vi "ActionVIOnCompile.vi"(8 "error in (no error)":errorcluster, 11 "Device Item Ref in":T1 format="%.0x") -> (0 "error out":errorcluster)   [LabVIEW 2019, in "OPC UA Client Addon System Explorer.lvlib"]
uses:
  OPC UA Client Addon System Explorer.lvlib
  <vilib>/NI VeriStand/Custom Device API/Custom Device Item Ref.ctl
  Addon Shared/Types/Tag.WriteProperties.Info.ctl
  <vilib>/NI VeriStand/Custom Device API/Data Reference.ctl
  Addon Shared/Types/Compiled.Settings.ctl
  Addon Shared/Types/OPCConnection.Properties.ctl
  Addon Shared/Types/Poll.ListProperties.ctl
  Addon Shared/Types/Tags.ReadWriteRefs.ctl
  <vilib>/NI VeriStand/Custom Device API/Custom Device Target Type.ctl
  <vilib>/NI VeriStand/Custom Device API/Data Access Type.ctl
  Addon Shared/Types/DataRefs.Location.ctl
  Addon Shared/SubVIs/Constants.vi
  <vilib>/NI VeriStand/Custom Device API/NI VeriStand - Get Item Property.vi
  <vilib>/NI VeriStand/Custom Device API/Get Item Property (String).vi
  <vilib>/NI VeriStand/Custom Device API/Get Item Property (U16).vi
  <vilib>/NI VeriStand/Custom Device API/Get Item Property (Dependent File).vi
  <vilib>/NI VeriStand/Custom Device API/Set Item Property (String).vi
  <vilib>/NI VeriStand/Custom Device API/Set Item Property (U16).vi
  <vilib>/Utility/libraryn.llb/Get File Extension.vi
  <vilib>/Utility/MD5Checksum.llb/MD5Checksum File.vi
  <vilib>/NI VeriStand/Custom Device API/Set Item Property (Dependent File).vi
  <vilib>/Utility/libraryn.llb/Check if File or Folder Exists.vi
  <vilib>/NI VeriStand/Custom Device API/NI VeriStand - Remove Item Property.vi
  <vilib>/NI VeriStand/Custom Device Tools/Custom Device Utility Library/NI VeriStand - Search for Item by GUID.vi
  <vilib>/NI VeriStand/Custom Device Tools/Custom Device Utility Library/NI VeriStand - Search for All Items by GUID.vi
  <vilib>/NI VeriStand/Custom Device API/Get Item Property (Dependent Node Pointer).vi
  <vilib>/NI VeriStand/Custom Device API/Set Item Property (U32).vi
  <vilib>/NI VeriStand/Custom Device API/Get Item Property (U32).vi
  <vilib>/NI VeriStand/Custom Device Tools/Custom Device Utility Library/NI VeriStand - Search for Item by Name.vi
  <vilib>/NI VeriStand/Custom Device API/Set Item Property (Variant).vi
  <vilib>/NI VeriStand/Custom Device Tools/Custom Device Utility Library/Custom Device Utility Library.lvlib
  Addon Shared/OPC UA Client Addon Shared.lvlib
  <vilib>/NI VeriStand/Custom Device API/Custom Device API.lvlib
  <vilib>/NI/NIVS Inline Async API/_Data Access System Explorer/Data Access System Explorer.lvlib
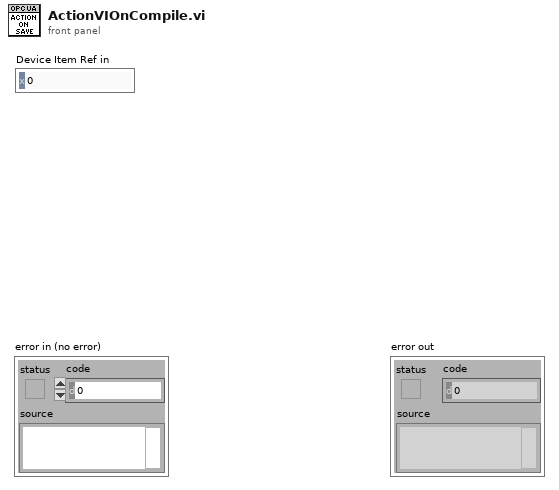
[diagram p1: front panel]
types:
  T1 = typedef "Custom Device API.lvlib/Custom Device Item Ref.ctl" = u64
  T2 = enum16{"Output/Write", "Input/Read", "Input/ReadWrite"}
  T3 = cluster{"Name":string, "Type":enum16{"Output/Write", "Input/Read", "Input/ReadWrite"}, "VS Refs":T1[]}
  T4 = typedef "OPC UA Client Addon Shared.lvlib/Tag.WriteProperties.Info.ctl" = cluster{"Path":string, "Offset":i32, "Length":i32, "DataType":u32}
  T5 = typedef "Custom Device API.lvlib/Data Reference.ctl" = i32
  T6 = typedef "OPC UA Client Addon Shared.lvlib/Compiled.Settings.ctl" = cluster{"Connection.Properties":T7, "PollEngine.Settings":T8[], "LUT":variant, "Write Locations":T4[], "TotalTags":u32, "Data Refs":T9, "Target Type":T10}
  T7 = typedef "OPC UA Client Addon Shared.lvlib/OPCConnection.Properties.ctl" = cluster{"Server IP Address":string, "Server Port":u16, "Message Mode":enum16{"None", "Sign", "Sign and Encrypt"}, "Security":enum16{"Basic256", "Basic128Rsa15"}, "User Name":string, "Password":string, "Client Certificate":path, "Server Certificate":path, "Server Certificate (RT)":path, "Client Certificate (RT)":path}
  T8 = typedef "OPC UA Client Addon Shared.lvlib/Poll.ListProperties.ctl" = cluster{"Poll Rate":dbl, "Tags":string[]}
  T9 = typedef "OPC UA Client Addon Shared.lvlib/Tags.ReadWriteRefs.ctl" = cluster{"Read Refs":T5[], "Read Values":dbl[], "Read?":bool[], "Access":enum8{"Null", "Read", "Write", "Read&Write"}[], "Write Refs":T5[], "Write Values":dbl[], "Write?":bool[], "Write Only Location":u32, "Write? Reset":bool[]}
  T10 = typedef "Custom Device API.lvlib/Custom Device Target Type.ctl" = enum16{"PharLap", "VxWorks", "Windows", "Linux_32_ARM", "Linux_x64"}
  T11 = typedef "Custom Device API.lvlib/Data Access Type.ctl" = enum16{"Read", "Write"}
  T12 = typedef "OPC UA Client Addon Shared.lvlib/DataRefs.Location.ctl" = cluster{"Offset":i32, "Length":i32}
  T13 = typedef "OPC UA Client Addon Shared.lvlib/Tag.Settings.ctl" = cluster{"TagPath":string, "DataType":u32, "DataAccess":u32}
  T14 = cluster{"Name":string, "Type":enum16{"Output/Write", "Input/Read", "Input/ReadWrite"}, "VS Refs":T1[]}[]
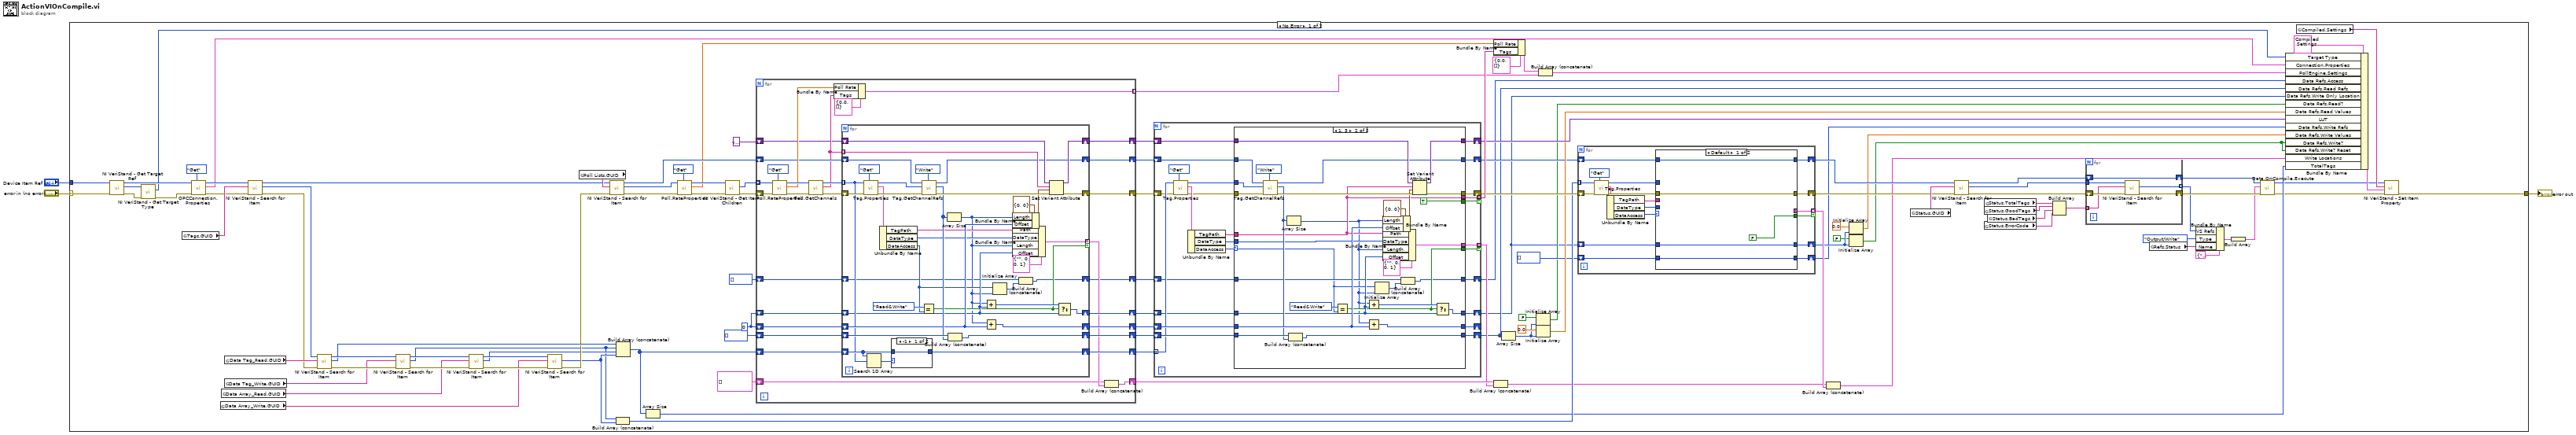
[diagram p0: block diagram]
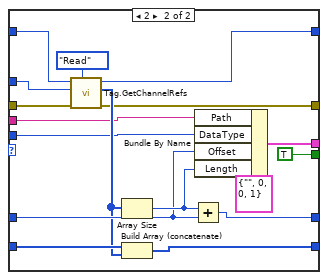
[diagram p2: hidden frame]
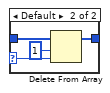
[diagram p4: hidden frame]
diagram:
  n1 = case shown="No Error" "error in (no error)" {
    selector: "error in (no error)" -> [w8 w295]
    tunnel: [w82 w295] -> w2
    tunnel: "Device Item Ref in" -> [w7 _]
    frame No Error {
      w43 = 0
      n2 = call <vilib>:"NI VeriStand - Get Target Ref.vi"("error in"=w8, "Item Ref in"=w7) -> ("error out"=w9:errorcluster, "Target Ref"=w10:T1, "Item Ref out"=w6:T1)  [unwired: 6 in, 1 out]
      n3 = call <vilib>:"NI VeriStand - Get Target Type.vi"("error in (no error)"=w9, "Item Ref in"=w10) -> ("error out"=w5:errorcluster, "Target Type"=w4:T10)  [unwired: 7 in, 1 out]
      n4 = global read "Constants.vi" "Tags.GUID"() -> (w103:string)
      n5 = call "OPCConnection.Properties.vi"("Action"=enum8{"Get", "Set"}."Get", "error in (no error)"=w5, "Item Ref in"=w6) -> ("error out"=w102:errorcluster, "Connection.Properties"=w83:T7, "Item Ref out"=w84:T1)  [unwired: 6 in]
      n6 = global read "Constants.vi" "Data Array_Write.GUID"() -> (w62:string)
      n7 = global read "Constants.vi" "Data Array_Read.GUID"() -> (w63:string)
      n8 = global read "Constants.vi" "Data Tag_Write.GUID"() -> (w96:string)
      n9 = global read "Constants.vi" "Data Tag_Read.GUID"() -> (w99:string)
      n10 = call-poly <vilib>:"NI VeriStand - Search for Item.vi"("error in"=w102, "Item GUID"=w103, "Section Ref in"=w84) -> ("error out"=w95:errorcluster, "Item Ref"=w100:T1, "Section Ref out"=w101:T1)  [unwired: 5 in, 1 out]
      n11 = call-poly <vilib>:"NI VeriStand - Search for Item.vi"("error in"=w95, "Item GUID"=w99, "Section Ref in"=w100) -> ("error out"=w97:errorcluster, "Item Refs"=w94:T1[], "Section Ref out"=w98:T1)  [unwired: 5 in, 1 out]
      n12 = call-poly <vilib>:"NI VeriStand - Search for Item.vi"("error in"=w97, "Item GUID"=w96, "Section Ref in"=w98) -> ("error out"=w66:errorcluster, "Item Refs"=w59:T1[], "Section Ref out"=w64:T1)  [unwired: 5 in, 1 out]
      n13 = call-poly <vilib>:"NI VeriStand - Search for Item.vi"("error in"=w66, "Item GUID"=w63, "Section Ref in"=w64) -> ("error out"=w68:errorcluster, "Item Refs"=w61:T1[], "Section Ref out"=w67:T1)  [unwired: 5 in, 1 out]
      n14 = call-poly <vilib>:"NI VeriStand - Search for Item.vi"("error in"=w68, "Item GUID"=w62, "Section Ref in"=w67) -> ("error out"=w65:errorcluster, "Item Refs"=w60:T1[])  [unwired: 5 in, 2 out]
      n15 = global read "Constants.vi" "Poll Lists.GUID"() -> (w111:string)
      n16 = call-poly <vilib>:"NI VeriStand - Search for Item.vi"("error in"=w65, "Item GUID"=w111, "Section Ref in"=w101) -> ("error out"=w110:errorcluster, "Item Ref"=w109:T1, "Section Ref out"=w93:T1)  [unwired: 5 in, 1 out]
      n17 = Build Array (concatenate)(w59, w60) -> (w57:T1[])
      n18 = Build Array (concatenate)(w94, w59, w61, w60) -> (w55:T1[])
      n19 = Array Size(array=w55) -> (size(s)=w54:i32)
      n20 = call "Poll.RateProperties.vi"("Action"=enum8{"Get", "Set"}."Get", "error in (no error)"=w110, "Item Ref in"=w109) -> ("error out"=w107:errorcluster, "Poll Rate"=w87:dbl, "Item Ref out"=w106:T1)  [unwired: 6 in]
      n21 = call <vilib>:"NI VeriStand - Get Item Children.vi"("error in (no error)"=w107, "Item Ref in"=w106) -> ("error out"=w105:errorcluster, "Child Refs"=w104:T1[])  [unwired: 6 in, 2 out]
      n22 = for {
        tunnel: w104 -> [w249] mode=indexing
        shift-right: [w245] -> w90
        shift-left: w55 -> [w246]
        shift-right: [w241] -> w89
        shift-left: w105 -> [w250]
        tunnel: [w238] -> w85 mode=indexing
        shift-right: [w236] -> w91
        shift-left: w93 -> [w240]
        shift-right: [w234] -> w70
        shift-left: variant ("variant") -> [w235]
        shift-right: [w232] -> w51
        shift-left: T5[] [] ("Array") -> [w233]
        shift-right: [w230] -> w50
        shift-left: w43 -> [w231]
        shift-right: [w228] -> w41
        shift-left: w43 -> [w229]
        shift-right: [w226] -> w40
        shift-left: T4[] [] -> [w225]
        shift-right: [w224] -> w29
        shift-left: u32[] [] -> [w223]
        n23 = call "Poll.RateProperties.vi"("Action"=enum8{"Get", "Set"}."Get", "error in (no error)"=w250, "Item Ref in"=w249) -> ("error out"=w248:errorcluster, "Poll Rate"=w244:dbl, "Item Ref out"=w247:T1)  [unwired: 6 in]
        n24 = call "Poll.GetChannels.vi"("error in (no error)"=w248, "Node Ptr"=w247) -> ("error out"=w242:errorcluster, "Tags"=w239:string[], "Refs"=w243:T1[])  [unwired: 7 in]
        n25 = Bundle By Name(cluster=T8 {"Poll Rate"=0.0, "Tags"=[]}, "Poll Rate"=w244, "Tags"=w239) -> (w238:T8)
        n26 = for {
          tunnel: w243 -> [w270] mode=indexing
          shift-right: [w288] -> w245
          shift-left: w246 -> [w287]
          shift-right: [w284] -> w241
          shift-left: w242 -> [w272]
          shift-right: [w281] -> w234
          shift-left: w235 -> [w283]
          tunnel: w239 -> [w282] mode=indexing
          shift-right: [w280] -> w236
          shift-left: w240 -> [w285]
          shift-right: [w278] -> w232
          shift-left: w233 -> [w279]
          shift-right: [w276] -> w230
          shift-left: w231 -> [w274]
          shift-right: [w260] -> w228
          shift-left: w229 -> [w261]
          tunnel: [w259] -> w227 mode=indexing if=w258
          shift-right: [w253] -> w224
          shift-left: w223 -> [w252]
          n27 = call "Tag.Properties.vi"("Action"=enum8{"Get", "Set"}."Get", "error in (no error)"=w272, "Section Ref in"=w270) -> ("error out"=w271:errorcluster, "Channel Settings"=w266:T13, "Item Ref out"=w269:T1)  [unwired: 6 in]
          n28 = Search 1D Array(1D array=w287, element=w270) -> (index of element=w289:i32)  [unwired: 1 in]
          n29 = Unbundle By Name(w266) -> ("TagPath"=w265:string, "DataType"=w264:u32, "DataAccess"=w256:u32)
          n30 = case shown="-1" w289 {
            selector: w289 -> [_ w293]
            tunnel: [w290 w291] -> w288
            tunnel: w287 -> [w290 w294]
            frame -1 {
            }
            frame Default {
              n31 = Delete From Array(array=w294, length=1, index=w293) -> (array with subset deleted=w291:T1[])  [unwired: 1 out]
            }
          }
          n32 = Equal?(x=enum16{"Null", "Read", "Write", "Read&Write"}."Read&Write" ("access"), y=w256) -> (x = y?=w258:bool)
          n33 = call "Tag.GetChannelRefs.vi"("Access"=Data_Access_Type."Write", "error in (no error)"=w271, "Dependent Node Ref"=w269, "Section Ref in"=w285) -> ("error out"=w286:errorcluster, "Array"=w277:T5[], "Section Ref out"=w280:T1)  [unwired: 5 in]
          n34 = Array Size(array=w277) -> (size(s)=w255:i32)
          n35 = Build Array (concatenate)(w279, w277) -> (w278:T5[])
          n36 = Add(x=w255, y=w261) -> (x+y=w262:i32)
          n37 = Add(x=w255, y=w274) -> (x+y=w276:i32)
          n38 = Initialize Array(w256, w255) -> (w254:u32[])
          n39 = Bundle By Name(cluster=T12 {"Offset"=0, "Length"=0}, "Length"=w255, "Offset"=w274) -> (w273:T12)
          n40 = Bundle By Name(cluster=T4 {"Path"="", "Offset"=0, "Length"=0, "DataType"=1} ("WriteData.Info"), "Path"=w265, "DataType"=w264, "Length"=w255, "Offset"=w261) -> (w259:T4)
          n41 = Build Array (concatenate)(w252, w254) -> (w253:u32[])
          n42 = Set Variant Attribute(Variant=w283, name=w282, value=w273, error in=w286) -> (Variant out=w281:variant, error out=w284:errorcluster)  [unwired: 1 out]
          n43 = Select(t=w262, s=w258, f=w261) -> (s? t:f=w260:i32)
        }
        n44 = Build Array (concatenate)(w225, w227) -> (w226:T4[])
      }
      n45 = for {
        shift-right: [w183] -> w58
        shift-left: w89 -> [w172]
        shift-right: [w181] -> w69
        shift-left: w70 -> [w182]
        tunnel: w90 -> [w174] mode=indexing
        shift-right: [w180] -> w47
        shift-left: w91 -> [w184]
        tunnel: [w166] -> w88 mode=indexing if=w179
        shift-right: [w176] -> _
        shift-left: w50 -> [w177]
        shift-right: [w175] -> w27
        shift-left: w51 -> [w178]
        shift-right: [w163] -> w22
        shift-left: w41 -> [w165]
        tunnel: [w162] -> w39 mode=indexing if=w161
        shift-right: [w159] -> w28
        shift-left: w29 -> [w160]
        n46 = call "Tag.Properties.vi"("Action"=enum8{"Get", "Set"}."Get", "error in (no error)"=w172, "Section Ref in"=w174) -> ("error out"=w170:errorcluster, "Channel Settings"=w171:T13, "Item Ref out"=w169:T1)  [unwired: 6 in]
        n47 = Unbundle By Name(w171) -> ("TagPath"=w167:string, "DataType"=w164:u32, "DataAccess"=w168:u32)
        n48 = case shown="1, 3" w168 {
          selector: w168 -> [_ w194]
          tunnel: w184 -> [w189 w216]
          tunnel: [w190 w222] -> w183
          tunnel: w182 -> [w191 w221]
          tunnel: [w191 w220] -> w181
          tunnel: [w189 w214] -> w180
          tunnel: w167 -> [_ w204]
          tunnel: w170 -> [w190 w218]
          tunnel: w169 -> [_ w215]
          tunnel: [_ TRUE] -> w179
          tunnel: w178 -> [w188 w212]
          tunnel: w177 -> [w187 w211]
          tunnel: [w187 w210] -> w176
          tunnel: [w188 w209] -> w175
          tunnel: [_ w204] -> w166
          tunnel: w165 -> [w186 w200]
          tunnel: w164 -> [_ w202]
          tunnel: [_ w199] -> w162
          tunnel: [w186 w198] -> w163
          tunnel: [_ w197] -> w161
          tunnel: w160 -> [w185 w195]
          tunnel: [w185 w193] -> w159
          frame Default {
          }
          frame 1, 3 {
            n49 = call "Tag.GetChannelRefs.vi"("Access"=Data_Access_Type."Write", "error in (no error)"=w218, "Dependent Node Ref"=w215, "Section Ref in"=w216) -> ("error out"=w217:errorcluster, "Array"=w208:T5[], "Section Ref out"=w214:T1)  [unwired: 5 in]
            n50 = Array Size(array=w208) -> (size(s)=w192:i32)
            n51 = Build Array (concatenate)(w212, w208) -> (w209:T5[])
            n52 = Equal?(x=enum16{"Null", "Read", "Write", "Read&Write"}."Read&Write" ("access"), y=w194) -> (x = y?=w197:bool)
            n53 = Add(x=w192, y=w200) -> (x+y=w201:i32)
            n54 = Add(x=w192, y=w211) -> (x+y=w210:i32)
            n55 = Initialize Array(w194, w192) -> (w196:u32[])
            n56 = Bundle By Name(cluster=T12 {"Offset"=0, "Length"=0}, "Length"=w192, "Offset"=w211) -> (w207:T12)
            n57 = Bundle By Name(cluster=T4 {"Path"="", "Offset"=0, "Length"=0, "DataType"=1} ("WriteData.Info"), "Path"=w204, "DataType"=w202, "Length"=w192, "Offset"=w200) -> (w199:T4)
            n58 = Build Array (concatenate)(w195, w196) -> (w193:u32[])
            n59 = Set Variant Attribute(Variant=w221, name=w204, value=w207, error in=w217) -> (Variant out=w220:variant, error out=w222:errorcluster)  [unwired: 1 out]
            n60 = Select(t=w201, s=w197, f=w200) -> (s? t:f=w198:i32)
          }
        }
      }
      n61 = Bundle By Name(cluster=T8 {"Poll Rate"=0.0, "Tags"=[]}, "Poll Rate"=w87, "Tags"=w88) -> (w86:T8)
      n62 = Build Array (concatenate)(w40, w39) -> (w23:T4[])
      n63 = Array Size(array=w27) -> (size(s)=w25:i32)
      n64 = Initialize Array(FALSE, w25) -> (w24:bool[])
      n65 = Initialize Array(0.0 ("element"), w25) -> (w48:dbl[])
      n66 = Build Array (concatenate)(w86, w85) -> (w32:T8[])
      n67 = for {
        tunnel: w57 -> [w120] mode=indexing
        shift-right: [w130] -> w45
        shift-left: w58 -> [w121]
        shift-right: [w129] -> w36
        shift-left: w22 -> [w128]
        tunnel: [w127] -> w38 mode=indexing if=w124
        shift-right: [w126] -> w31
        shift-left: T5[] [] ("Array") -> [w125]
        shift-right: [w122] -> w46
        shift-left: w47 -> [w123]
        n68 = call "Tag.Properties.vi"("Action"=enum8{"Get", "Set"}."Get", "error in (no error)"=w121, "Section Ref in"=w120) -> ("error out"=w118:errorcluster, "Channel Settings"=w116:T13, "Item Ref out"=w119:T1)  [unwired: 6 in]
        n69 = Unbundle By Name(w116) -> ("TagPath"=w114:string, "DataType"=w115:u32, "DataAccess"=w113:u32)
        n70 = case shown="Default" w113 {
          tunnel: [w133 w143] -> w130
          tunnel: [w134 w152] -> w129
          tunnel: w128 -> [w134 w150]
          tunnel: [_ w149] -> w127
          tunnel: [w135 w148] -> w126
          tunnel: w125 -> [w135 w147]
          tunnel: w118 -> [w133 w139]
          tunnel: w119 -> [_ w136]
          tunnel: [FALSE TRUE] -> w124
          tunnel: w123 -> [w131 w145]
          tunnel: [w131 w142] -> w122
          tunnel: w115 -> [_ w138]
          tunnel: w114 -> [_ w137]
          frame Default {
          }
          frame 2 {
            n71 = call "Tag.GetChannelRefs.vi"("Access"=Data_Access_Type."Read", "error in (no error)"=w139, "Dependent Node Ref"=w136, "Section Ref in"=w145) -> ("error out"=w143:errorcluster, "Array"=w144:T5[], "Section Ref out"=w142:T1)  [unwired: 5 in]
            n72 = Array Size(array=w144) -> (size(s)=w151:i32)
            n73 = Build Array (concatenate)(w147, w144) -> (w148:T5[])
            n74 = Add(x=w151, y=w150) -> (x+y=w152:i32)
            n75 = Bundle By Name(cluster=T4 {"Path"="", "Offset"=0, "Length"=0, "DataType"=1} ("WriteData.Info"), "Path"=w137, "DataType"=w138, "Offset"=w150, "Length"=w151) -> (w149:T4)
          }
        }
      }
      n76 = Build Array (concatenate)(w23, w38) -> (w33:T4[])
      n77 = Initialize Array(0.0 ("element"), w36) -> (w34:dbl[])
      n78 = Initialize Array(FALSE, w36) -> (w21:bool[])
      n79 = global read "Constants.vi" "Status.GUID"() -> (w78:string)
      n80 = call-poly <vilib>:"NI VeriStand - Search for Item.vi"("error in"=w45, "Item GUID"=w78, "Section Ref in"=w46) -> ("error out"=w76:errorcluster, "Item Ref"=w77:T1, "Section Ref out"=w56:T1)  [unwired: 5 in, 1 out]
      n81 = global read "Constants.vi" "Status.GoodTags"() -> (w74:string)
      n82 = global read "Constants.vi" "Status.ErrorCode"() -> (w53:string)
      n83 = global read "Constants.vi" "Status.TotalTags"() -> (w75:string)
      n84 = global read "Constants.vi" "Status.BadTags"() -> (w73:string)
      n85 = Build Array(w75, w74, w73, w53) -> (w72:string[])
      n86 = for {
        tunnel: w77 -> [w158]
        shift-right: [w154] -> w20
        shift-left: w76 -> [w157]
        tunnel: w72 -> [w156] mode=indexing
        tunnel: [w153] -> w15 mode=indexing
        shift-right: [w155] -> w18
        shift-left: w56 -> [w155]
        n87 = call-poly <vilib>:"NI VeriStand - Search for Item.vi"("error in"=w157, "Item Name"=w156, "Section Ref in"=w158) -> ("error out"=w154:errorcluster, "Item Ref"=w153:T1)  [unwired: 5 in, 2 out]
      }
      n88 = global read "Constants.vi" "Refs.Status"() -> (w13:string)
      n89 = Bundle By Name(cluster=T3 {"Name"="", "Type"=enum."Output/Write", "VS Refs"=[]} ("Group"), "VS Refs"=w15, "Type"=T2."Output/Write", "Name"=w13) -> (w12:T3)
      n90 = Build Array(w12) -> (w11:T14)
      n91 = call <vilib>:"Data.OnCompile.Execute.vi"("error in"=w20, "VS Ref Groups"=w11, "Custom Device Ref"=w18) -> ("error out"=w19:errorcluster, "Custom Device Ref"=w17:T1)  [unwired: 7 in]
      n92 = Bundle By Name(cluster=T6 {"Connection.Properties"={"Server IP Address"="", "Server Port"=0, "Message Mode"=enum."None", "Security"=enum."Basic256", "User Name"="", "Password"="", "Client Certificate"=path "", "Server Certificate"=path "", "Server Certificate (RT)"=path "", "Client Certificate (RT)"=path ""}, "PollEngine.Settings"=[], "LUT"=variant, "Write Locations"=[], "TotalTags"=0, "Data Refs"={"Read Refs"=[], "Read Values"=[], "Read?"=[], "Access"=[], "Write Refs"=[], "Write Values"=[], "Write?"=[], "Write Only Location"=0, "Write? Reset"=[]}, "Target Type"=enum."PharLap"}, "Target Type"=w4, "Connection.Properties"=w83, "PollEngine.Settings"=w32, "Data Refs.Access"=w28, "Data Refs.Read Refs"=w27, "Data Refs.Write Only Location"=w22, "Data Refs.Read?"=w24, "Data Refs.Read Values"=w48, "LUT"=w69, "Data Refs.Write Refs"=w31, "Data Refs.Write Values"=w34, "Data Refs.Write?"=w21, "Data Refs.Write? Reset"=w21, "Write Locations"=w33, "TotalTags"=w54) -> (w81:T6)
      n93 = global read "Constants.vi" "Compiled.Settings"() -> (w80:string)
      n94 = call-poly <vilib>:"NI VeriStand - Set Item Property.vi"("error in (no error)"=w19, "Value"=w81, "Property Name"=w80, "Item Ref in"=w17) -> ("error out"=w82:errorcluster)  [unwired: 5 in, 2 out]
    }
    frame Error {
    }
  }
  "error out" <- w2
